vi "[FPGA] PID Float Simple Multichannel 00.vi"(4 "Auto/Manual":bool=TRUE, 6 "reinitialize? (F)":bool, 8 "Channel Config.":T1={"Write Channel"=FALSE, "Channel #"=0, "dt (s)"=2.5e-06, "Kp"=10.0, "Ki [Hz]"=5000.0, "Kd [Hz]"=500.0, "upper limit"=32768.0, "lower limit"=-32768.0, "LPF alpha"=0.07283} {"Kp" step=0.125}, 9 "Channel #":u32, 10 "Process Variable":sgl, 11 "Setpoint":sgl) -> (0 "dt out (s)":sgl, 1 "Enabled":bool, 3 "Output":sgl)   [LabVIEW 2015]
uses:
  Controls/PID Float Simple Multichannel Channel Configuration.ctl
  Controls/PID State.ctl
  <vilib>/rvi/DataTransferAndStorage/Container/Common/niFpgaContainerGetUniqueNameForEmu.vi
  <vilib>/rvi/DataTransferAndStorage/Container/Common/niFpgaContainerSetEmuInfo.vi
  <vilib>/rvi/eio/common/nirviEmuReportErrorAndStop.vi
  <vilib>/rvi/DataTransferAndStorage/Container/Common/niFpgaContainerExecOnDevCompGetState.vi
  <vilib>/rvi/Emulation/niFpgaEmulationIsFPGAContextNoSignature.vi
  <vilib>/rvi/Emulation/niFpgaProcessEmulError.vi
  <vilib>/rvi/Emulation/niFpgaSctlEmulationGetInTimedLoop.vi
  <vilib>/rvi/errors/nirviReportUnexpectedCaseInternalError (U32).vi
  <vilib>/rvi/Memory/Memory_Emulation/niFpgaMemoryEmulationCacheClearOnFirstRun.vi
  <vilib>/rvi/Memory/Memory_Emulation/nirvimemoryEmulationManagerCache_MakeExclusive.vi
  <vilib>/rvi/Memory/Memory_Emulation/niFpgaMemoryEmulationValidateCache.vi
  <vilib>/rvi/Memory/Memory_Emulation/nirvimemoryEmulationManagerCache_InsertValue.vi
  <vilib>/Utility/error.llb/Clear Errors.vi
  <vilib>/rvi/Memory/Memory_Emulation/nirvimemoryEmulationManagerCache_ReleaseExclusive.vi
  <vilib>/rvi/Memory/Memory_Emulation/nirvimemoryEmulationManagerCache_GetValue.vi
  <vilib>/rvi/Memory/Memory_Emulation/nirvimemoryEmulationManagerCache_SetValue.vi
  <vilib>/rvi/Emulation/niFpgaSctlEmulationResourceMgr.vi
  Floating Point/Polymorphic subVIs/Multiply 00.vi
  Floating Point/Polymorphic subVIs/Subtract 00.vi
  Floating Point/Polymorphic subVIs/Divide 00.vi
  Floating Point/Polymorphic subVIs/Add 00.vi
  <vilib>/rvi/LocalResourceManager/LocalResourceManager.xnode
  <vilib>/rvi/DataTransferAndStorage/Container/XNode/niFpgaContainer.xnode
  <vilib>/rvi/Memory/Memory_Emulation/niFpgaMemoryEmulationRefIn.vi
panel:
  out "Bumpless":bool
  in  "Manual Output":sgl
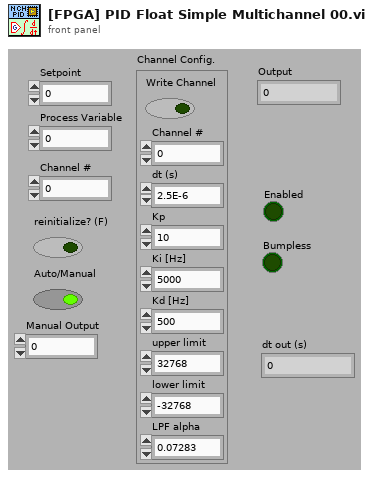
[diagram p1: front panel]
types:
  T1 = typedef "PID Float Simple Multichannel Channel Configuration.ctl" = cluster{"Write Channel":bool, "Channel #":u32, "dt (s)":sgl, "Kp":sgl, "Ki [Hz]":sgl, "Kd [Hz]":sgl, "upper limit":sgl, "lower limit":sgl, "LPF alpha":sgl}
  T2 = typedef "PID State.ctl" = cluster{"uI(k-1)":sgl, "e(k-1)":sgl, "fPV(k-1)":sgl, "Output (k-1)":sgl}
  T3 = cluster{"Write Channel":bool, "Channel #":u32, "dt (s)":sgl, "Kp":sgl, "Ki [Hz]":sgl, "Kd [Hz]":sgl, "upper limit":sgl, "lower limit":sgl, "LPF alpha":sgl}
  T4 = cluster{"uI(k-1)":sgl, "e(k-1)":sgl, "fPV(k-1)":sgl, "Output (k-1)":sgl}
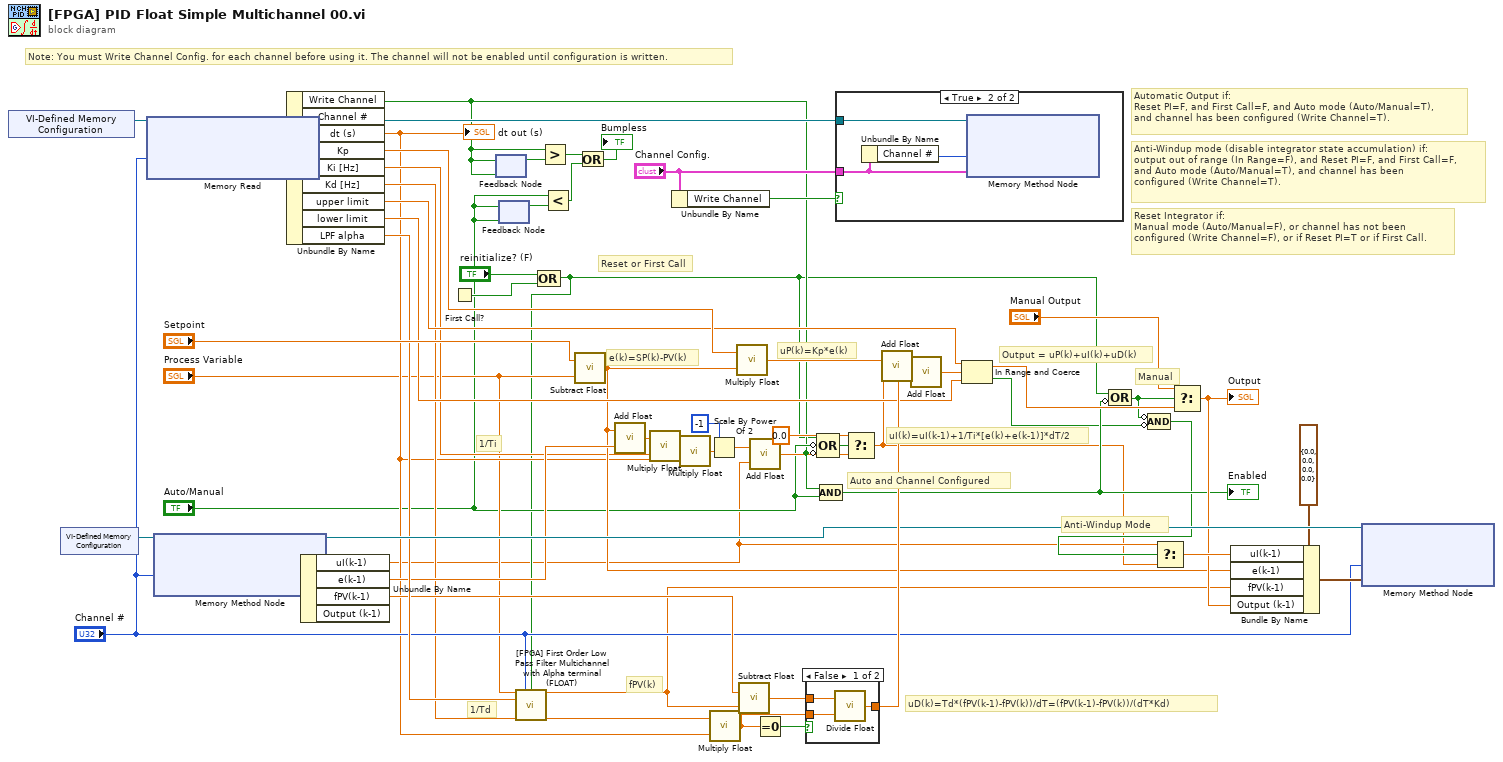
[diagram p0: block diagram]
diagram:
  # "Anti-Windup Mode"
  # "Manual"
  # "Auto and Channel Configured"
  # "Reset or First Call"
  # "Automatic Output if:\nReset PI=F, and First Call=F, and Auto mode (Auto/Manual=T),\nand channel has been configured (Write Channel=T)."
  # "Anti-Windup mode (disable integrator state accumulation) if: \noutput out of range (In Range=F), and Reset PI=F, and First Call=F,\nand Auto mode (Auto/Manual=T), and channel has been \nconfigured (Write Channel=T)."
  # "Reset Integrator if: \nManual mode (Auto/Manual=F), or channel has not been \nconfigured (Write Channel=F), or if Reset PI=T or if First Call."
  # "1/Td"
  # "Note: You must Write Channel Config. for each channel before using it. The channel will not be enabled until configuration is written."
  # "uP(k)=Kp*e(k)"
  # "1/Ti"
  # "fPV(k)"
  # "uD(k)=Td*(fPV(k-1)-fPV(k))/dT=(fPV(k-1)-fPV(k))/(dT*Kd)"
  # "uI(k)=uI(k-1)+1/Ti*[e(k)+e(k-1)]*dT/2"
  # "e(k)=SP(k)-PV(k)"
  # "Output = uP(k)+uI(k)+uD(k)"
  n1 = xnode ("VI-Defined Memory Configuration")() -> ("Memory Out"=w47:refnum<k21>)
  n2 = xnode ("VI-Defined Memory Configuration")() -> ("Memory Out"=w48:refnum<k21>)
  n3 = xnode ("Memory Read")("Address"="Channel #", "Memory In"=w47) -> ("Data"=w45:T3, "Memory Out"=w46:refnum<k21>)
  n4 = xnode ("Memory Method Node")("Address"="Channel #", "Memory In"=w48) -> ("Data"=w40:T4, "Memory Out"=w49:refnum<k21>)
  n5 = Unbundle By Name(w45) -> ("Write Channel"=w11:bool, "dt (s)"=w22:sgl, "Kp"=w44:sgl, "Ki [Hz]"=w29:sgl, "Kd [Hz]"=w23:sgl, "upper limit"=w43:sgl, "lower limit"=w42:sgl, "LPF alpha"=w41:sgl)  [unwired: 1 out]
  "dt out (s)" <- w22
  n6 = Unbundle By Name(w40) -> ("uI(k-1)"=w3:sgl, "e(k-1)"=w34:sgl, "fPV(k-1)"=w35:sgl)  [unwired: 1 out]
  n7 = First Call?() -> (First Call?: T/F=w27:bool)
  n8 = feedback-in #1(w11) -> ()
  n9 = feedback #1(w11) -> (w17:bool)
  n10 = feedback #2("Auto/Manual") -> (w15:bool)
  n11 = feedback-in #2("Auto/Manual") -> ()
  n12 = Compound Arithmetic op=OR("reinitialize? (F)", w27) -> (w7:bool)
  n13 = call "[FPGA] First Order Low Pass Filter Multichannel with Alpha terminal (FLOAT).vi"("x"="Process Variable", "Channel #"="Channel #", "reset"=w7, "LPF alpha"=w41) -> ("filtered x"=w19:sgl)  [unwired: 11 in]
  n14 = Greater?(x=w11, y=w17) -> (0:w16:bool)
  n15 = Less?(x="Auto/Manual", y=w15) -> (x < y?=w14:bool)
  n16 = call-poly "Subtract Float.vi"("y"="Process Variable", "x"="Setpoint") -> ("x*y"=w33:sgl)
  n17 = Or(x=w16, y=w14) -> (x .or. y?=→"Bumpless":bool)
  n18 = call-poly "Add Float.vi"("y"=w34, "x"=w33) -> ("x+y"=w53:sgl)
  n19 = call-poly "Multiply Float.vi"("y"=w29, "x"=w53) -> ("x*y"=w54:sgl)
  n20 = Unbundle By Name("Channel Config.") -> ("Write Channel"=w26:bool)
  n21 = call-poly "Multiply Float.vi"("y"=w22, "x"=w54) -> ("x*y"=w52:sgl)
  n22 = Scale By Power Of 2(n=i16 -1, x=w52) -> (x*2^n=w51:sgl)
  n23 = call-poly "Multiply Float.vi"("y"=w22, "x"=w23) -> ("x*y"=w21:sgl)
  n24 = call-poly "Multiply Float.vi"("y"=w33, "x"=w44) -> ("x*y"=w32:sgl)
  n25 = call-poly "Subtract Float.vi"("y"=w19, "x"=w35) -> ("x*y"=w24:sgl)
  n26 = call-poly "Add Float.vi"("y"=w3, "x"=w51) -> ("x+y"=w58:sgl)
  n27 = Equal To 0?(x=w21) -> (x = 0?=w20:bool)
  n28 = case shown="False" w20 {
    tunnel: [w62 _] -> w50
    tunnel: w24 -> [w61 _]
    tunnel: w21 -> [w60 _]
    frame False {
      n29 = call-poly "Divide Float.vi"("y"=w60, "x"=w61) -> ("x/y"=w62:sgl)
    }
    frame True {
    }
  }
  n30 = Compound Arithmetic op=OR(w7, invert "Auto/Manual", invert w11) -> (w1:bool)
  n31 = Compound Arithmetic op=AND(w11, "Auto/Manual") -> (w8:bool)
  "Enabled" <- w8
  n32 = case shown="True" w26 {
    tunnel: w46 -> [_ w65]
    tunnel: "Channel Config." -> [_ w64]
    frame False {
    }
    frame True {
      n33 = Unbundle By Name(w64) -> ("Channel #"=w63:u32)
      n34 = xnode ("Memory Method Node")("Address"=w63, "Data"=w64, "Memory In"=w65) -> ()  [unwired: 1 out]
    }
  }
  n35 = Select(t=sgl 0.0, s=w1, f=w58) -> (s? t:f=w2:sgl)
  n36 = call-poly "Add Float.vi"("y"=w2, "x"=w32) -> ("x+y"=w56:sgl)
  n37 = call-poly "Add Float.vi"("y"=w50, "x"=w56) -> ("x+y"=w31:sgl)
  n38 = In Range and Coerce(upper limit=w43, x=w31, lower limit=w42) -> (coerced(x)=w9:sgl, In Range?=w6:bool)
  n39 = Compound Arithmetic op=OR(w7, invert w8) -> (w5:bool)
  n40 = Compound Arithmetic op=AND(invert w5, invert w6) -> (w4:bool)
  n41 = Select(t=w3, s=w4, f=w2) -> (s? t:f=w37:sgl)
  n42 = Select(t="Manual Output", s=w5, f=w9) -> (s? t:f=w36:sgl)
  "Output" <- w36
  n43 = Bundle By Name(cluster=T2 {"uI(k-1)"=0.0, "e(k-1)"=0.0, "fPV(k-1)"=0.0, "Output (k-1)"=0.0} ("State"), "uI(k-1)"=w37, "e(k-1)"=w33, "fPV(k-1)"=w19, "Output (k-1)"=w36) -> (w38:T2)
  n44 = xnode ("Memory Method Node")("Address"="Channel #", "Data"=w38, "Memory In"=w49) -> ()  [unwired: 1 out]
